vi "PodControlCostFunctionCore.vi"(8 "Cost Function Weights":T1, 9 "Linear Speed":dbl, 10 "Output States":T2, 11 "Coerrected Timestep":dbl) -> (2 "All States Out":T1, 3 "Cost":dbl)   [LabVIEW 2014]
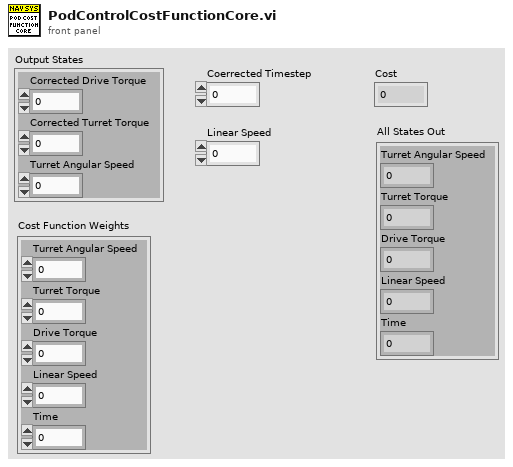
[diagram p1: front panel]
types:
  T1 = cluster{"Turret Angular Speed":dbl, "Turret Torque":dbl, "Drive Torque":dbl, "Linear Speed":dbl, "Time":dbl}
  T2 = cluster{"Corrected Drive Torque":dbl, "Corrected Turret Torque":dbl, "Turret Angular Speed":dbl}
  T3 = cluster{"Corrected Drive Torque":dbl, "Corrected Turret Torque":dbl, "Turret Angular Speed":dbl, "Linear Speed":dbl, "Coerrected Timestep":dbl}
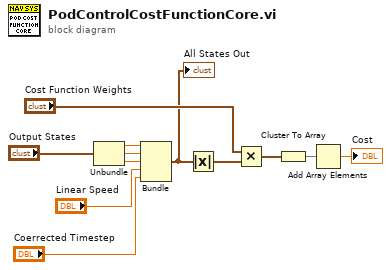
[diagram p0: block diagram]
diagram:
  n1 = Unbundle("Output States") -> ("Corrected Drive Torque"=w11:dbl, "Corrected Turret Torque"=w10:dbl, "Turret Angular Speed"=w9:dbl)
  n2 = Bundle("Corrected Drive Torque"=w11, "Corrected Turret Torque"=w10, "Turret Angular Speed"=w9, "Linear Speed"="Linear Speed", "Coerrected Timestep"="Coerrected Timestep") -> (w4:T3)  [unwired: 1 in]
  "All States Out" <- w4
  n3 = Absolute Value(x=w4) -> (abs(x)=w6:T3)
  n4 = Multiply(x="Cost Function Weights", y=w6) -> (x*y=w3:cluster{dbl, dbl, dbl, "Linear Speed":dbl, dbl})
  n5 = Cluster To Array(cluster=w3) -> (array=w2:dbl[])
  n6 = Add Array Elements(numeric array=w2) -> (sum=→"Cost":dbl)
